vi "VALVE_change_position.vi"(3 "error in":errorcluster, 4 "valve positions":cluster{"Valve H":u8, "OldVal":u8}, 5 "VISA valve":refnum<visa-resource-name>) -> (0 "error out":errorcluster, 1 "Valve position OUT":u8, 2 "Valve error":bool)   [LabVIEW 2015]
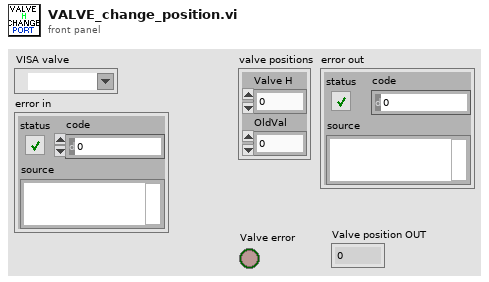
[diagram p1: front panel]
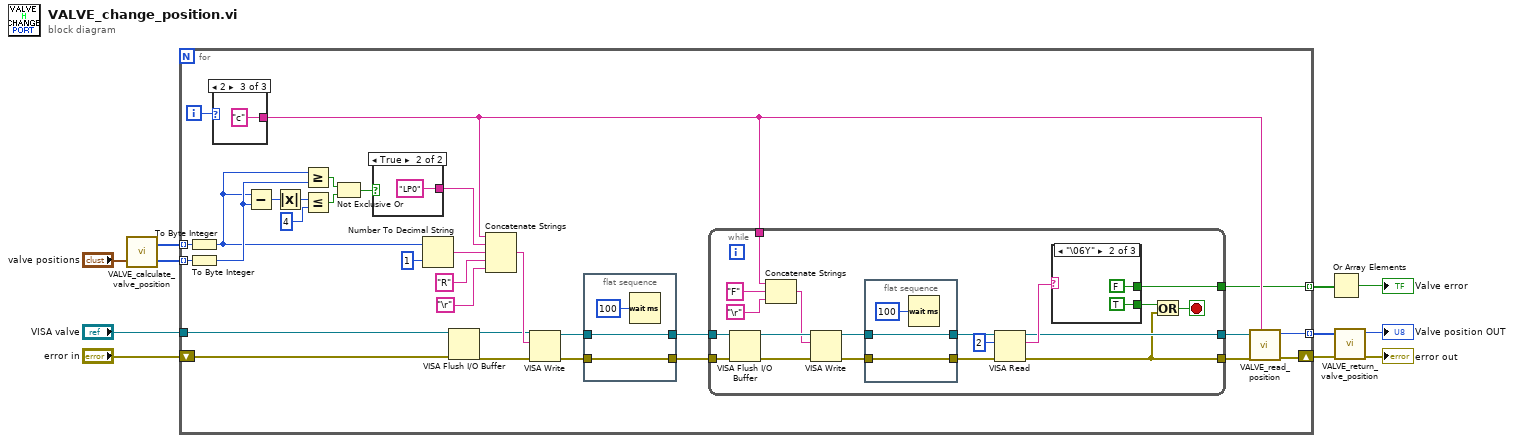
[diagram p0: block diagram]
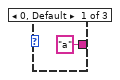
[diagram p2: hidden frame]
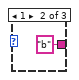
[diagram p3: hidden frame]
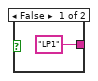
[diagram p4: hidden frame]
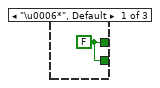
[diagram p5: hidden frame]
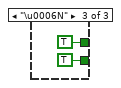
[diagram p6: hidden frame]
diagram:
  n1 = call "VALVE_calculate_valve_position.vi"("valve positions"="valve positions") -> ("Valves positions Old"=w7:u8[], "Valves positions New"=w8:u8[])  [unwired: 1 in]
  n2 = for {
    tunnel: "VISA valve" -> [w30]
    shift-right: [w13] -> w6
    shift-left: "error in" -> [w29]
    tunnel: w8 -> [w27] mode=indexing
    tunnel: w7 -> [w26] mode=indexing
    tunnel: [w14] -> w4 mode=indexing
    tunnel: [w12] -> w2 mode=indexing
    i -> [w28]
    n3 = To Byte Integer(number=w27) -> (8bit integer=w18:i8)
    n4 = To Byte Integer(number=w26) -> (8bit integer=w22:i8)
    n5 = case shown="2" w28 {
      tunnel: ["a" "b" "c"] -> w15
      frame 0, Default {
      }
      frame 1 {
      }
      frame 2 {
      }
    }
    n6 = Subtract(x=w18, y=w22) -> (x-y=w25:i8)
    n7 = Absolute Value(x=w25) -> (abs(x)=w24:i8)
    n8 = Greater Or Equal?(x=w18, y=w22) -> (x >= y?=w21:bool)
    n9 = Less Or Equal?(x=w24, y=i8 4) -> (x <= y?=w20:bool)
    n10 = Not Exclusive Or(1:w20, 2:w21) -> (0:w19:bool)
    n11 = case shown="True" w19 {
      tunnel: ["LP1" ("buffer d'écriture") "LP0" ("buffer d'écriture")] -> w31
      frame False {
      }
      frame True {
      }
    }
    n12 = Number To Decimal String(number=w18, width (-)=i16 1) -> (decimal integer string=w40:string)
    n13 = VISA Flush I/O Buffer(VISA resource name=w30, error in (no error)=w29) -> (VISA resource name out=w36:refnum<visa-resource-name>, error out=w37:errorcluster)  [unwired: 1 in]
    n14 = Concatenate Strings(w15, w31, w40, "R" ("string"), "\r") -> (w39:string)
    n15 = VISA Write(VISA resource name=w36, write buffer=w39, error in (no error)=w37) -> (VISA resource name out=w35:refnum<visa-resource-name>, error out=w33:errorcluster)  [unwired: 1 out]
    n16 = flat-sequence {
      tunnel: w35 -> [w77]
      tunnel: [w77] -> w34
      tunnel: w33 -> [w76]
      tunnel: [w76] -> w32
      frame #0 {
        n17 = Wait (ms)(milliseconds to wait=u32 100) -> ()  [unwired: 1 out]
      }
    }
    n18 = while {
      tunnel: w32 -> [w60]
      tunnel: w34 -> [w59]
      tunnel: [w49] -> w16
      tunnel: [w53] -> w17
      tunnel: w15 -> [w52]
      tunnel: [w48] -> w12
      stop <- w51 stop-if-true
      n19 = VISA Flush I/O Buffer(VISA resource name=w59, error in (no error)=w60) -> (VISA resource name out=w58:refnum<visa-resource-name>, error out=w57:errorcluster)  [unwired: 1 in]
      n20 = Concatenate Strings(w52, "F" ("string"), "\r") -> (w55:string)
      n21 = VISA Write(VISA resource name=w58, write buffer=w55, error in (no error)=w57) -> (VISA resource name out=w62:refnum<visa-resource-name>, error out=w63:errorcluster)  [unwired: 1 out]
      n22 = flat-sequence {
        tunnel: w62 -> [w74]
        tunnel: [w74] -> w64
        tunnel: w63 -> [w73]
        tunnel: [w73] -> w65
        frame #0 {
          n23 = Wait (ms)(milliseconds to wait=u32 100) -> ()  [unwired: 1 out]
        }
      }
      n24 = VISA Read(VISA resource name=w64, byte count=u32 2, error in (no error)=w65) -> (VISA resource name out=w53:refnum<visa-resource-name>, read buffer=w54:string, error out=w49:errorcluster)  [unwired: 1 out]
      n25 = case shown="\"\\06Y\"" w54 {
        tunnel: [w67 FALSE TRUE] -> w48
        tunnel: [w67 TRUE TRUE] -> w50
        frame "\u0006*", Default {
          w67 = FALSE
        }
        frame "\u0006Y" {
        }
        frame "\u0006N" {
        }
      }
      n26 = Or(x=w50, y=w49) -> (x .or. y?=w51:bool)
    }
    n27 = call "VALVE_read_position.vi"("Valve adress"=w15, "error in"=w16, "VISA valve"=w17) -> ("error out"=w13:errorcluster, "Valve position OUT"=w14:u8)  [unwired: 4 in]
  }
  n28 = Or Array Elements(Boolean array=w2) -> (logical OR=→"Valve error":bool)
  n29 = call "VALVE_return_valve_position.vi"("error in"=w6, "Valves positions"=w4) -> ("error out"=→"error out":errorcluster, "Position"=→"Valve position OUT":u8)  [unwired: 4 in]
